vi "DeltaE(CMC).vi"(1 "l:c":bool, 2 "L*a*b colors":T1) -> (0 "Delta E":dbl)   [LabVIEW 2013]
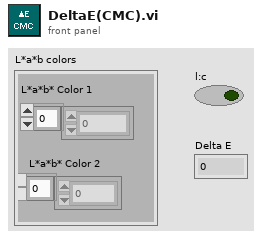
[diagram p1: front panel]
types:
  T1 = cluster{"L*a*b* Color 1":dbl[], "L*a*b* Color 2":dbl[]}
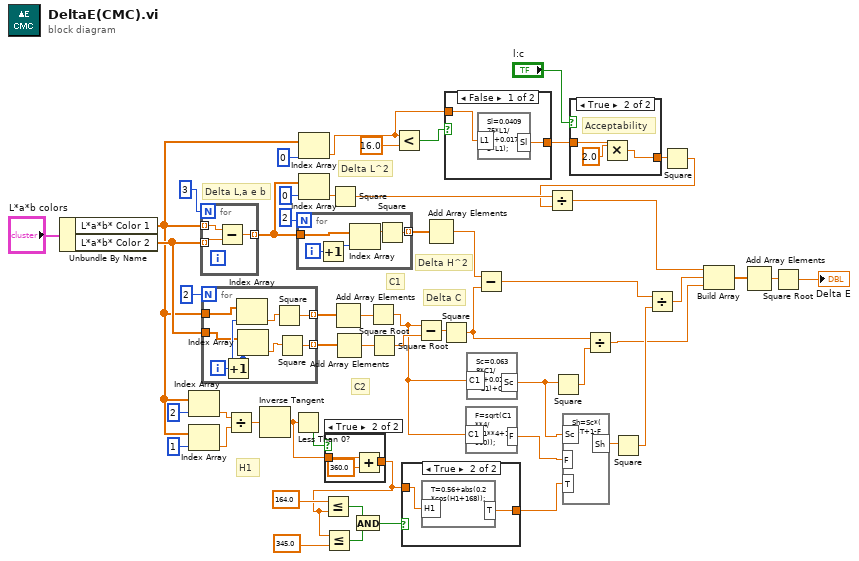
[diagram p0: block diagram]
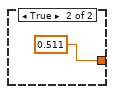
[diagram p3: hidden frame]
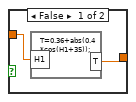
[diagram p5: hidden frame]
diagram:
  # "Delta L^2"
  # "H1"
  # "Delta H^2"
  # "Delta C"
  # "C2"
  # "C1"
  # "Delta L,a e b"
  n1 = Unbundle By Name("L*a*b colors") -> ("L*a*b* Color 1"=w22:dbl[], "L*a*b* Color 2"=w51:dbl[])
  n2 = Index Array(array=w22, index=2) -> (element=w36:dbl)
  n3 = Index Array(array=w22, index=1) -> (element=w35:dbl)
  n4 = for {
    N: 3 -> [_]
    tunnel: w22 -> [w57] mode=indexing
    tunnel: w51 -> [w56] mode=indexing
    tunnel: [w55] -> w41 mode=indexing
    n5 = Subtract(x=w57, y=w56) -> (x-y=w55:dbl)
  }
  n6 = for {
    N: 2 -> [_]
    tunnel: w22 -> [w64]
    tunnel: w51 -> [w62]
    tunnel: [w59] -> w50 mode=indexing
    tunnel: [w58] -> w49 mode=indexing
    i -> [w65]
    n7 = Increment(x=w65) -> (x+1=w63:i32)
    n8 = Index Array(array=w64, index=w63) -> (element=w61:dbl)
    n9 = Index Array(array=w62, index=w63) -> (element=w60:dbl)
    n10 = Square(x=w61) -> (x^2=w59:dbl)
    n11 = Square(x=w60) -> (x^2=w58:dbl)
  }
  n12 = Divide(x=w36, y=w35) -> (x/y=w34:dbl)
  n13 = Inverse Tangent(1:w34) -> (0:w27:dbl)
  n14 = Less Than 0?(x=w27) -> (x < 0?=w28:bool)
  n15 = for {
    N: 2 -> [_]
    tunnel: w41 -> [w69]
    tunnel: [w66] -> w44 mode=indexing
    i -> [w70]
    n16 = Increment(x=w70) -> (x+1=w68:i32)
    n17 = Index Array(array=w69, index=w68) -> (element=w67:dbl)
    n18 = Square(x=w67) -> (x^2=w66:dbl)
  }
  n19 = Index Array(array=w22, index=0) -> (element=w18:dbl)
  n20 = Index Array(array=w41, index=0) -> (element=w39:dbl)
  n21 = case shown="True" w28 {
    tunnel: w27 -> [w71 w74]
    tunnel: [w71 w72] -> w26
    frame False {
    }
    frame True {
      n22 = Add(x=w74, y=360.0) -> (x+y=w72:dbl)
    }
  }
  n23 = Less Or Equal?(x=164.0, y=w26) -> (x <= y?=w30:bool)
  n24 = Less Or Equal?(x=w26, y=345.0 ("x")) -> (x <= y?=w31:bool)
  n25 = Square(x=w39) -> (x^2=w12:dbl)
  n26 = Add Array Elements(numeric array=w50) -> (sum=w48:dbl)
  n27 = Add Array Elements(numeric array=w49) -> (sum=w47:dbl)
  n28 = And(x=w30, y=w31) -> (x .and. y?=w29:bool)
  n29 = Square Root(x=w48) -> (sqrt(x)=w25:dbl)
  n30 = Square Root(x=w47) -> (sqrt(x)=w46:dbl)
  n31 = Less?(x=w18, y=16.0) -> (x < y?=w19:bool)
  n32 = case shown="True" w29 {
    tunnel: w26 -> [w76 w78]
    tunnel: [w75 w77] -> w23
    frame False {
      n33 = formula code="T=0.36+abs(0.4*cos(H1+35));"("H1"=w76) -> ("T"=w75:dbl)
    }
    frame True {
      n34 = formula code="T=0.56+abs(0.2*cos(H1+168));"("H1"=w78) -> ("T"=w77:dbl)
    }
  }
  n35 = Subtract(x=w25, y=w46) -> (x-y=w43:dbl)
  n36 = Add Array Elements(numeric array=w44) -> (sum=w42:dbl)
  n37 = Square(x=w43) -> (x^2=w9:dbl)
  n38 = case shown="False" w19 {
    tunnel: [w79 0.511] -> w16
    tunnel: w18 -> [w80 _]
    frame False {
      n39 = formula code="Sl=0.040975*L1/(1+0.01765*L1);"("L1"=w80) -> ("Sl"=w79:dbl)
    }
    frame True {
    }
  }
  n40 = formula code="F=sqrt(C1**4/(C1**4+1900));"("C1"=w25) -> ("F"=w24:dbl)
  n41 = formula code="Sc=0.0638*C1/(1+0.0131*C1)+0.638;"("C1"=w25) -> ("Sc"=w13:dbl)
  n42 = Subtract(x=w42, y=w9) -> (x-y=w7:dbl)
  n43 = Square(x=w13) -> (x^2=w10:dbl)
  n44 = formula code="Sh=Sc*(F*T+1-F);"("Sc"=w13, "F"=w24, "T"=w23) -> ("Sh"=w14:dbl)
  n45 = case shown="True" "l:c" {
    tunnel: w16 -> [w82 w85]
    tunnel: [w82 w83] -> w15
    frame False {
      # "Perceptibily"
    }
    frame True {
      # "Acceptability"
      n46 = Multiply(x=2.0, y=w85) -> (x*y=w83:dbl)
    }
  }
  n47 = Divide(x=w9, y=w10) -> (x/y=w4:dbl)
  n48 = Square(x=w14) -> (x^2=w8:dbl)
  n49 = Divide(x=w7, y=w8) -> (x/y=w5:dbl)
  n50 = Square(x=w15) -> (x^2=w11:dbl)
  n51 = Divide(x=w12, y=w11) -> (x/y=w6:dbl)
  n52 = Build Array(w6, w5, w4) -> (w3:dbl[])
  n53 = Add Array Elements(numeric array=w3) -> (sum=w2:dbl)
  n54 = Square Root(x=w2) -> (sqrt(x)=→"Delta E":dbl)
